vi "Get Image.vi"(8 "error in":errorcluster, 9 "Reset Stats?":bool, 10 "Calc Stats?":bool, 11 "Camera Imaqdx in":refnum<class "Camera Imaqdx.lvclass">) -> (0 "error out":errorcluster, 2 "Image out":T1, 3 "Camera Imaqdx out":refnum<class "Camera Imaqdx.lvclass">)   [LabVIEW 2023, in "Camera Imaqdx.lvclass"]
uses:
  Camera Imaqdx.lvclass
  Camera Imaqdx.lvclass/Camera Imaqdx.ctl
  Camera Base/Camera Base.lvclass
  Camera Base/Acquisition Stats.ctl
  E:/git/HAL/Camera Base/Camera Base.lvclass
  E:/git/HAL/Hardware_class/Instrument.lvclass
  E:/git/HAL/Interfaces/ICamera/ICamera.lvclass
  E:/git/HAL/Camera Imaqdx/Camera Imaqdx.lvclass
  <vilib>/vision/Image Controls.llb/IMAQ Image.ctl
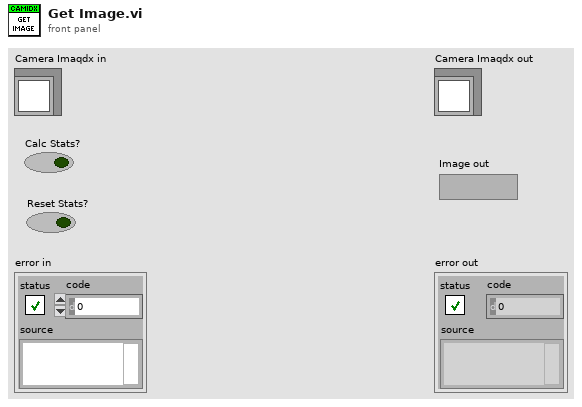
[diagram p1: front panel]
types:
  T1 = typedef "IMAQ Image.ctl" = refnum<image>
  T2 = typedef "IMAQdx.ctl" = refnum<k21>
  T3 = typedef "Camera Base.lvclass/Acquisition Stats.ctl" = cluster{"Acquired FPS":dbl, "Processed FPS":dbl, "Images Behind":u32, "Images Missed":u32}
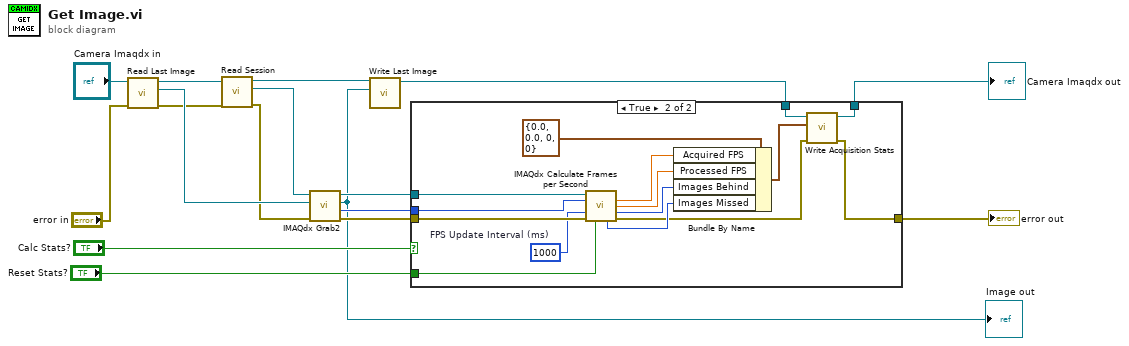
[diagram p0: block diagram]
diagram:
  n1 = call-dynamic "Read Last Image.vi"("error in (no error)"="error in", "Camera Base in"="Camera Imaqdx in") -> ("error out"=w2:errorcluster, "Image"=w7:T1, "Camera Base out"=w4:refnum<class "Camera Imaqdx.lvclass">)  [unwired: 7 in]
  n2 = call "Read Session.vi"("error in (no error)"=w2, "Camera Imaqdx in"=w4) -> ("error out"=w1:errorcluster, "IMAQdx Session"=w16:T2, "Camera Imaqdx out"=w3:refnum<class "Camera Imaqdx.lvclass">)  [unwired: 7 in]
  n3 = call <vilib>:"IMAQdx Grab2.vi"("error in"=w1, "Image In"=w7, "Session In"=w16) -> ("error out"=w14:errorcluster, "Buffer Number Out"=w13:u32, "Image Out"=w6:T1, "Session Out"=w15:T2)  [unwired: 5 in]
  "Image out" <- w6
  n4 = call-dynamic "Write Last Image.vi"("Image"=w6, "Camera Base in"=w3) -> ("Camera Base out"=w5:refnum<class "Camera Imaqdx.lvclass">)  [unwired: 8 in, 1 out]
  n5 = case shown="True" "Calc Stats?" {
    tunnel: w15 -> [_ w34]
    tunnel: w14 -> [w19 w33]
    tunnel: w13 -> [_ w32]
    tunnel: [w19 w21] -> w12
    tunnel: "Reset Stats?" -> [_ w31]
    tunnel: w5 -> [w18 w29]
    tunnel: [w18 w20] -> w10
    frame False {
    }
    frame True {
      w30 = u32 1000  # FPS Update Interval (ms)
      n6 = call <vilib>:"IMAQdx Calculate Frames per Second.vi"("Session In"=w34, "Buffer Number"=w32, "Frames per Second Update Interval (ms)"=w30, "error in (no error)"=w33, "Reset Counters"=w31) -> ("Acquired Frames per Second"=w27:dbl, "Processed Frames per Second"=w26:dbl, "Images Behind"=w25:i32, "Images Missed"=w24:u32, "error out"=w22:errorcluster)  [unwired: 4 in, 2 out]
      n7 = Bundle By Name(cluster=T3 {"Acquired FPS"=0.0, "Processed FPS"=0.0, "Images Behind"=0, "Images Missed"=0} ("Acquisition Stats"), "Acquired FPS"=w27, "Processed FPS"=w26, "Images Behind"=w25, "Images Missed"=w24) -> (w23:T3)
      n8 = call "Write Acquisition Stats.vi"("error in (no error)"=w22, "Acquisition Stats"=w23, "Camera Base in"=w29) -> ("error out"=w21:errorcluster, "Camera Base in"=w20:refnum<class "Camera Imaqdx.lvclass">)  [unwired: 7 in]
    }
  }
  "error out" <- w12
  "Camera Imaqdx out" <- w10
